vi "故障告警分析.vi"(8 "告警代码":u16, 9 "故障代码":u16, 10 "运行步序":u16, 11 "参数":string) -> (2 "报警内容":T1, 3 "简易报警状态":cluster{"故障状态":string, "报警状态":string})   [LabVIEW 2016, in "斯坦道总氮V2.lvlib"]
panel:
  # "1、注射泵水样阀口堵塞；\n2、注射泵阀过载或丝杆无动作。"
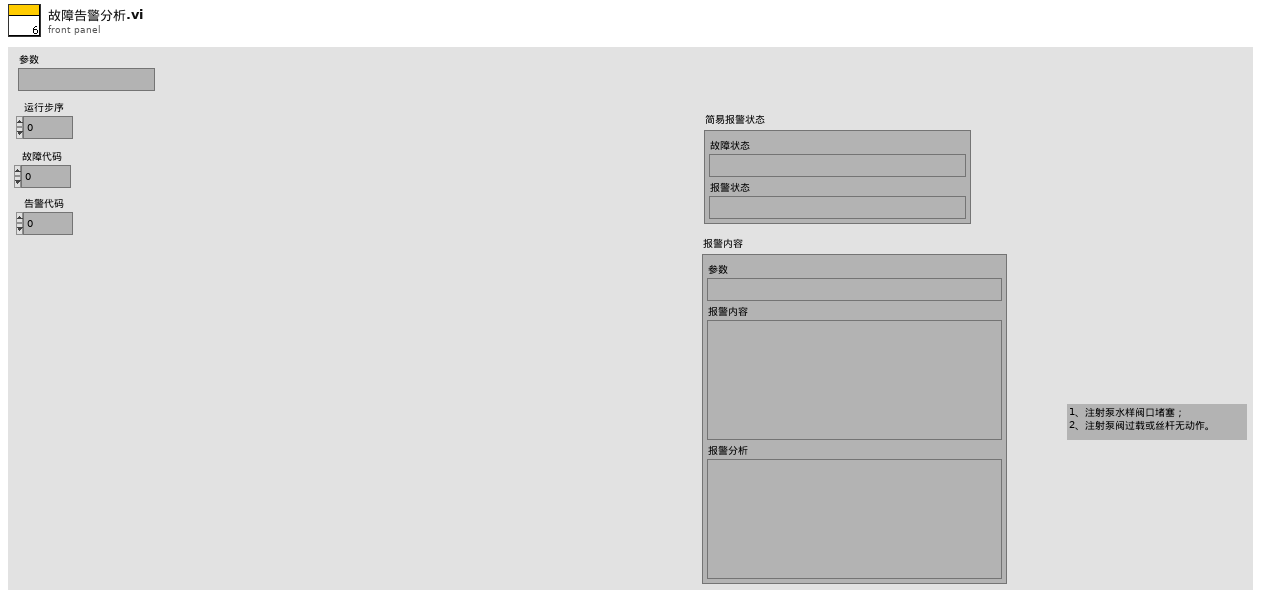
[diagram p1: front panel]
types:
  T1 = cluster{"参数":string, "报警内容":string, "报警分析":string}
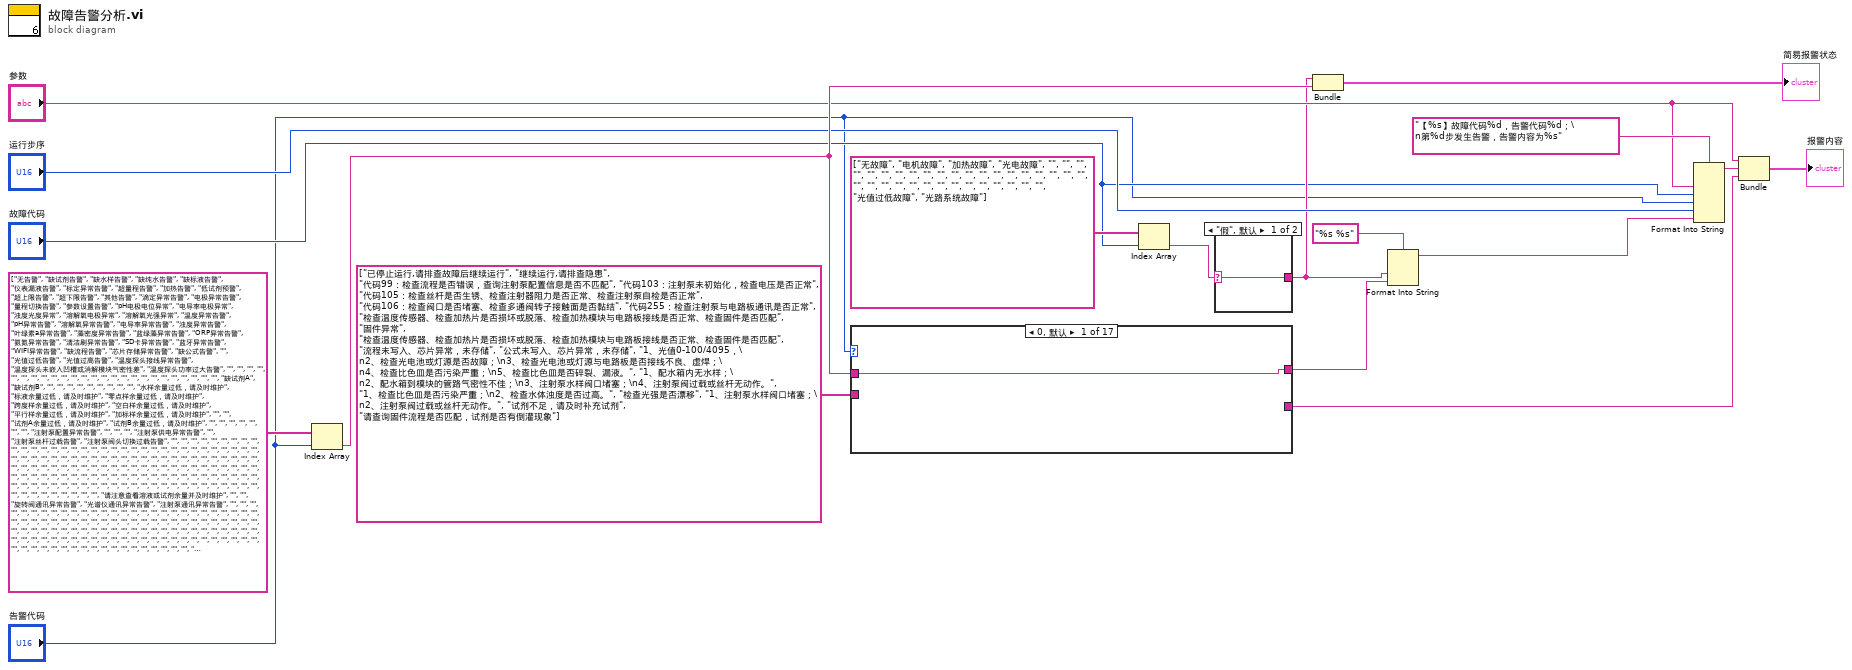
[diagram p0: block diagram]
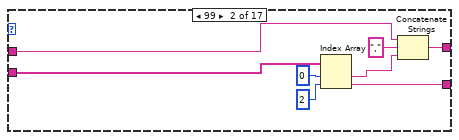
[diagram p3: hidden frame]
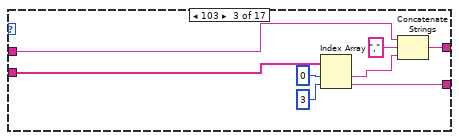
[diagram p4: hidden frame]
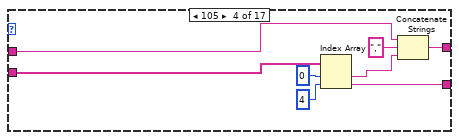
[diagram p5: hidden frame]
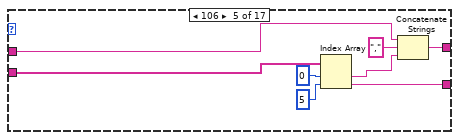
[diagram p6: hidden frame]
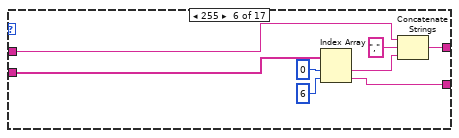
[diagram p7: hidden frame]
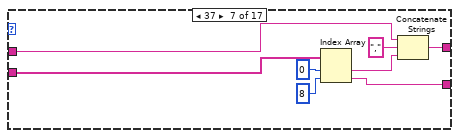
[diagram p8: hidden frame]
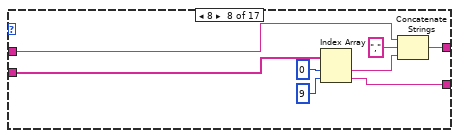
[diagram p9: hidden frame]
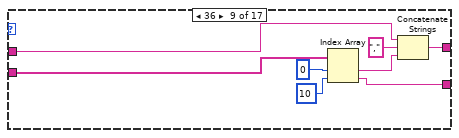
[diagram p10: hidden frame]
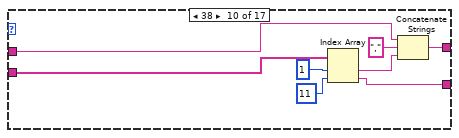
[diagram p11: hidden frame]
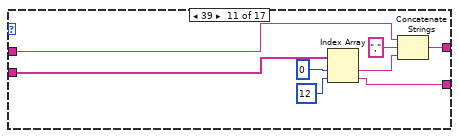
[diagram p12: hidden frame]
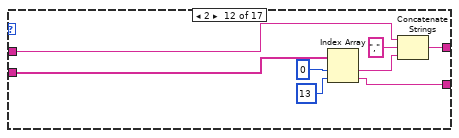
[diagram p13: hidden frame]
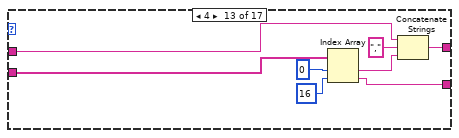
[diagram p14: hidden frame]
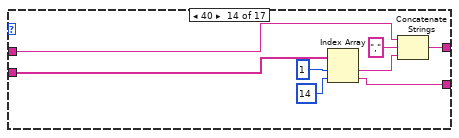
[diagram p15: hidden frame]
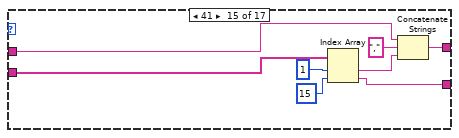
[diagram p16: hidden frame]
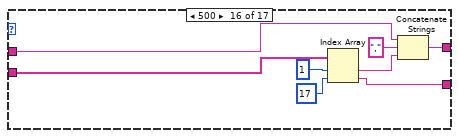
[diagram p17: hidden frame]
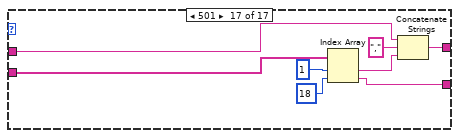
[diagram p18: hidden frame]
diagram:
  n1 = Index Array(array=string[] ["无告警", "缺试剂告警", "缺水样告警", "缺纯水告警", "缺标液告警", "仪表漏液告警", "标定异常告警", "超量程告警", "加热告警", "低试剂预警", "超上限告警", "超下限告警", "其他告警", "滴定异常告警", "电极异常告警", "量程切换告警", "参数设置告警", "pH电极电位异常", "电导率电极异常", "浊度光度异常", "溶解氧电极异常", "溶解氧光强异常", "温度异常告警", "pH异常告警", "溶解氧异常告警", "电导率异常告警", "浊度异常告警", "叶绿素a异常告警", "藻密度异常告警", "蓝绿藻异常告警", "ORP异常告警", "氨氮异常告警", "清洁刷异常告警", "SD卡异常告警", "蓝牙异常告警", "WIFI异常告警", "缺流程告警", "芯片存储异常告警", "缺公式告警", "", "光值过低告警", "光值过高告警", "温度探头接线异常告警", "温度探头未嵌入凹槽或消解模块气密性差", "温度探头功率过大告警", "", "", "", "", "", "", "", "", "", "", "", "", "", "", "", "", "", "", "", "", "", "", "", "", "", "缺试剂A", "缺试剂B", "", "", "", "", "", "", "", "", "", "水样余量过低，请及时维护", "标液余量过低，请及时维护", "零点样余量过低，请及时维护", "跨度样余量过低，请及时维护", "空白样余量过低，请及时维护", "平行样余量过低，请及时维护", "加标样余量过低，请及时维护", "", "", "试剂A余量过低，请及时维护", "试剂B余量过低，请及时维护", "", "", "", "", "", "", "", "注射泵配置异常告警", "", "", "", "注射泵供电异常告警", "", "注射泵丝杆过载告警", "注射泵阀头切换过载告警", "", "", "", "", "", "", "", "", "", "", "", "", "", "", "", "", "", "", "", "", "", "", "", "", "", "", "", "", "", "", "", "", "", "", "", "", "", "", "", "", "", "", "", "", "", "", "", "", "", "", "", "", "", "", "", "", "", "", "", "", "", "", "", "", "", "", "", "", "", "", "", "", "", "", "", "", "", "", "", "", "", "", "", "", "", "", "", "", "", "", "", "", "", "", "", "", "", "", "", "", "", "", "", "", "", "", "", "", "", "", "", "", "", "", "", "", "", "", "", "", "", "", "", "", "", "", "", "", "", "", "", "", "", "", "", "", "", "", "", "", "", "", "", "请注意查看溶液或试剂余量并及时维护", "", "", "旋转阀通讯异常告警", "光谱仪通讯异常告警", "注射泵通讯异常告警", "", "", "", "", "", "", "", "", "", "", "", "", "", "", "", "", "", "", "", "", "", "", "", "", "", "", "", "", "", "", "", "", "", "", "", "", "", "", "", "", "", "", "", "", "", "", "", "", "", "", "", "", "", "", "", "", "", "", "", "", "", "", "", "", "", "", "", "", "", "", "", "", "", "", "", "", "", "", "", "", "", "", "", "", "", "", "", "", "", "", "", "", "", "", "", "", "", "", "", "", "", "", "", "", "", "", "", "", "", "", "", "", "", "", "", "", "", "", "", "", "", "", "", "", "", "", "", "", "", "", "", "", "", "", "", "", "", "", "", "", "", "", "", "", "", "", "", "", "", "", "", "", "", "", "", "", "", "", "", "", "", "", "", "", "", "", "", "", "", "", "", "", "", "", "", "", "", "", "", "", "", "", "", "", "", "", "", "", "", "", "", "", "", "", "", "", "", "", "", "", "", "", "", "", "", "", "", "", "", "", "", "", "", "", "", "", "", "", "", "", "", "", "", "", "", "", "", "", "", "", "", "", "", "", "", "", "", "", "", "", "", "", "", "", "试剂不足", "试剂余量检测异常"], index="告警代码") -> (element=w14:string)
  n2 = case shown="0, 默认" "告警代码" {
    tunnel: string[] ["已停止运行,请排查故障后继续运行", "继续运行,请排查隐患", "代码99：检查流程是否错误，查询注射泵配置信息是否不匹配", "代码103：注射泵未初始化，检查电压是否正常", "代码105：检查丝杆是否生锈、检查注射器阻力是否正常、检查注射泵自检是否正常", "代码106：检查阀口是否堵塞、检查多通阀转子接触面是否黏结", "代码255：检查注射泵与电路板通讯是否正常", "检查温度传感器、检查加热片是否损坏或脱落、检查加热模块与电路板接线是否正常、检查固件是否匹配", "固件异常", "检查温度传感器、检查加热片是否损坏或脱落、检查加热模块与电路板接线是否正常、检查固件是否匹配", "流程未写入、芯片异常，未存储", "公式未写入、芯片异常，未存储", "1、光值0-100/4095，\n2、检查光电池或灯源是否故障；\n3、检查光电池或灯源与电路板是否接线不良、虚焊；\n4、检查比色皿是否污染严重；\n5、检查比色皿是否碎裂、漏液。", "1、配水箱内无水样；\n2、配水箱到模块的管路气密性不佳；\n3、注射泵水样阀口堵塞；\n4、注射泵阀过载或丝杆无动作。", "1、检查比色皿是否污染严重；\n2、检查水体浊度是否过高。", "检查光强是否漂移", "1、注射泵水样阀口堵塞；\n2、注射泵阀过载或丝杆无动作。", "试剂不足，请及时补充试剂", "请查询固件流程是否匹配，试剂是否有倒灌现象"] -> [_ w27 w35 w43 w51 w59 w67 w75 w83 w91 w99 w107 w115 w123 w131 w139 w147]
    tunnel: [w19 w22 w30 w38 w46 w54 w62 w70 w78 w86 w94 w102 w110 w118 w126 w134 w142] -> w6
    tunnel: [_ w23 w31 w39 w47 w55 w63 w71 w79 w87 w95 w103 w111 w119 w127 w135 w143] -> w12
    tunnel: w14 -> [w19 w21 w29 w37 w45 w53 w61 w69 w77 w85 w93 w101 w109 w117 w125 w133 w141]
    frame 0, Default {
    }
    frame 99 {
      n3 = Index Array(array=w27, index #1=0 ("索引"), index #2=2 ("索引")) -> (element #1=w25:string, element #2=w23:string)
      n4 = Concatenate Strings(w21, "," ("字符串"), w25) -> (w22:string)
    }
    frame 103 {
      n5 = Index Array(array=w35, index #1=0 ("索引"), index #2=3 ("索引")) -> (element #1=w33:string, element #2=w31:string)
      n6 = Concatenate Strings(w29, "," ("字符串"), w33) -> (w30:string)
    }
    frame 105 {
      n7 = Index Array(array=w43, index #1=0 ("索引"), index #2=4 ("索引")) -> (element #1=w41:string, element #2=w39:string)
      n8 = Concatenate Strings(w37, "," ("字符串"), w41) -> (w38:string)
    }
    frame 106 {
      n9 = Index Array(array=w51, index #1=0 ("索引"), index #2=5 ("索引")) -> (element #1=w49:string, element #2=w47:string)
      n10 = Concatenate Strings(w45, "," ("字符串"), w49) -> (w46:string)
    }
    frame 255 {
      n11 = Index Array(array=w59, index #1=0 ("索引"), index #2=6 ("索引")) -> (element #1=w57:string, element #2=w55:string)
      n12 = Concatenate Strings(w53, "," ("字符串"), w57) -> (w54:string)
    }
    frame 37 {
      n13 = Index Array(array=w67, index #1=0 ("索引"), index #2=8 ("索引")) -> (element #1=w65:string, element #2=w63:string)
      n14 = Concatenate Strings(w61, "," ("字符串"), w65) -> (w62:string)
    }
    frame 8 {
      n15 = Index Array(array=w75, index #1=0 ("索引"), index #2=9 ("索引")) -> (element #1=w73:string, element #2=w71:string)
      n16 = Concatenate Strings(w69, "," ("字符串"), w73) -> (w70:string)
    }
    frame 36 {
      n17 = Index Array(array=w83, index #1=0 ("索引"), index #2=10 ("索引")) -> (element #1=w81:string, element #2=w79:string)
      n18 = Concatenate Strings(w77, "," ("字符串"), w81) -> (w78:string)
    }
    frame 38 {
      n19 = Index Array(array=w91, index #1=1 ("索引"), index #2=11 ("索引")) -> (element #1=w89:string, element #2=w87:string)
      n20 = Concatenate Strings(w85, "," ("字符串"), w89) -> (w86:string)
    }
    frame 39 {
      n21 = Index Array(array=w99, index #1=0 ("索引"), index #2=12 ("索引")) -> (element #1=w97:string, element #2=w95:string)
      n22 = Concatenate Strings(w93, "," ("字符串"), w97) -> (w94:string)
    }
    frame 2 {
      n23 = Index Array(array=w107, index #1=0 ("索引"), index #2=13 ("索引")) -> (element #1=w105:string, element #2=w103:string)
      n24 = Concatenate Strings(w101, "," ("字符串"), w105) -> (w102:string)
    }
    frame 4 {
      n25 = Index Array(array=w115, index #1=0 ("索引"), index #2=16 ("索引")) -> (element #1=w113:string, element #2=w111:string)
      n26 = Concatenate Strings(w109, "," ("字符串"), w113) -> (w110:string)
    }
    frame 40 {
      n27 = Index Array(array=w123, index #1=1 ("索引"), index #2=14 ("索引")) -> (element #1=w121:string, element #2=w119:string)
      n28 = Concatenate Strings(w117, "," ("字符串"), w121) -> (w118:string)
    }
    frame 41 {
      n29 = Index Array(array=w131, index #1=1 ("索引"), index #2=15 ("索引")) -> (element #1=w129:string, element #2=w127:string)
      n30 = Concatenate Strings(w125, "," ("字符串"), w129) -> (w126:string)
    }
    frame 500 {
      n31 = Index Array(array=w139, index #1=1 ("索引"), index #2=17 ("索引")) -> (element #1=w137:string, element #2=w135:string)
      n32 = Concatenate Strings(w133, "," ("字符串"), w137) -> (w134:string)
    }
    frame 501 {
      n33 = Index Array(array=w147, index #1=1 ("索引"), index #2=18 ("索引")) -> (element #1=w145:string, element #2=w143:string)
      n34 = Concatenate Strings(w141, "," ("字符串"), w145) -> (w142:string)
    }
  }
  n35 = Index Array(array=string[] ["无故障", "电机故障", "加热故障", "光电故障", "", "", "", "", "", "", "", "", "", "", "", "", "", "", "", "", "", "", "", "", "", "", "", "", "", "", "", "", "", "", "", "", "", "", "光值过低故障", "光路系统故障"], index="故障代码") -> (element=w17:string)
  n36 = case shown="\"假\", 默认" w17 {
    selector: w17 -> [w148 _]
    tunnel: [w148 _] -> w5
    frame "假", Default {
    }
    frame "无故障" {
    }
  }
  n37 = Bundle(w5, w14) -> (→"简易报警状态":cluster{string, string})  [unwired: 1 in]
  n38 = Format Into String(format string="%s %s" ("格式字符串"), w5, w6) -> (resulting string=w7:string)  [unwired: 2 in, 1 out]
  n39 = Format Into String(format string="【%s】故障代码%d，告警代码%d；\n第%d步发生告警，告警内容为%s" ("格式字符串"), "参数", "故障代码", "告警代码", "运行步序", w7) -> (resulting string=w3:string)  [unwired: 2 in, 1 out]
  n40 = Bundle("参数"="参数", w3, w12) -> (→"报警内容":cluster{"参数":string, string, string})  [unwired: 1 in]
